vi "Clear Lookup Table.vi"(8 "error in (no error)":errorcluster, 11 "LookupTable Reference":refnum<data-value>) -> (0 "error out":errorcluster, 3 "LookupTable Reference Out":refnum<data-value>)   [LabVIEW 2020, in "MVA Framework.lvlib" / "LookupTable.lvlib" / "LookupTable.lvclass"]
doc: "清除查找表"
uses:
  LookupTable.lvclass
  LookupTable.lvclass/LookupTable.ctl
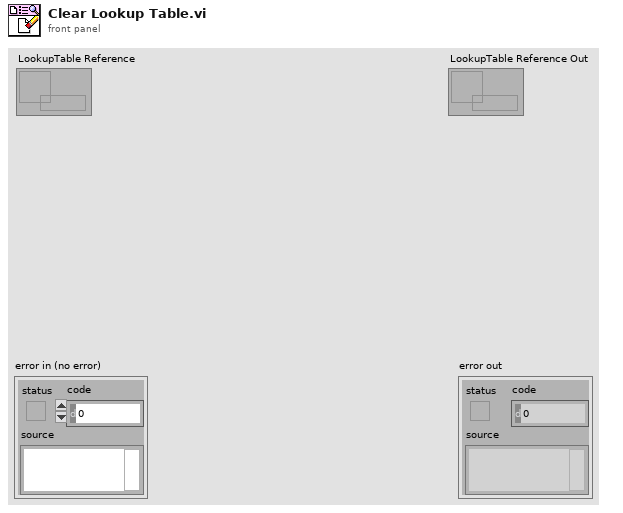
[diagram p1: front panel]
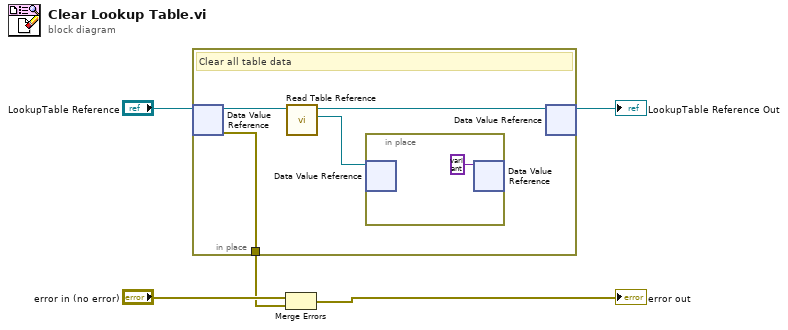
[diagram p0: block diagram]
diagram:
  n1 = in-place {
    in-place-border: [w9] -> w1
    # "Clear all table data"
    n2 = in-place-dvr #1("LookupTable Reference") -> (w8:refnum<class "LookupTable.lvclass">, w9:errorcluster)
    n3 = call "Read Table Reference.vi"("LookupTable in"=w8) -> ("Table Reference"=w7:refnum<data-value>, "LookupTable out"=w6:refnum<class "LookupTable.lvclass">)  [unwired: 9 in]
    n4 = in-place {
      n5 = in-place-dvr #2(w7) -> ()  [unwired: 2 out]
      n6 = in-place-dvr #2(variant ("data value")) -> ()  [unwired: 2 out]
    }
    n7 = in-place-dvr #1(w6) -> (→"LookupTable Reference Out":refnum<data-value>)  [unwired: 1 out]
  }
  n8 = Merge Errors("error in (no error)", w1) -> (→"error out":errorcluster)
